vi "Close.vi"(8 "error in (no error)":errorcluster, 11 "Arduino Detector in":refnum<class "Arduino Detector.lvclass">) -> (0 "error out":errorcluster, 3 "Arduino Detector out":refnum<class "Arduino Detector.lvclass">)   [LabVIEW 2019, in "Arduino Detector.lvclass"]
uses:
  Arduino Detector.lvclass
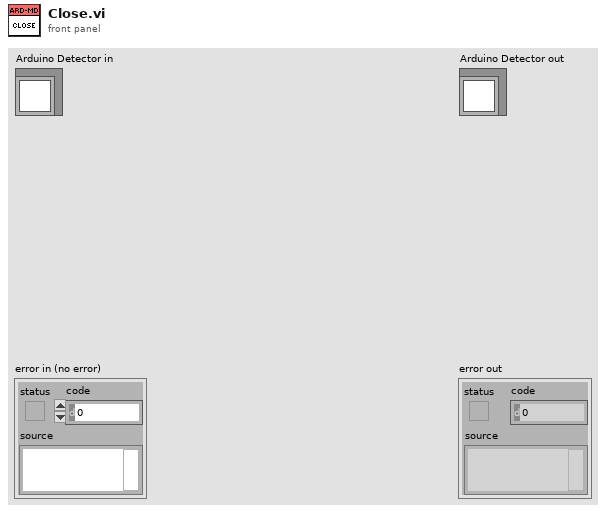
[diagram p1: front panel]
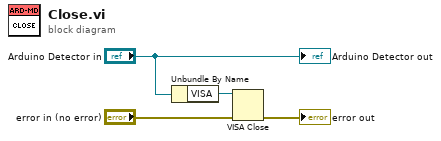
[diagram p0: block diagram]
diagram:
  n1 = Unbundle By Name("Arduino Detector in") -> ("VISA"=w1:refnum<visa-resource-name>)
  n2 = VISA Close(VISA resource name=w1, error in (no error)="error in (no error)") -> (error out=→"error out":errorcluster)
  "Arduino Detector out" <- "Arduino Detector in"
